vi "Pulse_Sequence_Global.vi"() -> ()   [LabVIEW 2021]
uses:
  Drivers/Arduino_Pulse_Generator/Configurate/Channel_Pulse_Stream.ctl
panel:
  out "Init outp register 2 (8-13)":bool[](array[boolean])
  out "Init outp register 1 (2-7)":bool[](array[boolean])
  out "Pulse sequence":T1[](array[typedef]) {"channel" min=2 max=13 step=1}
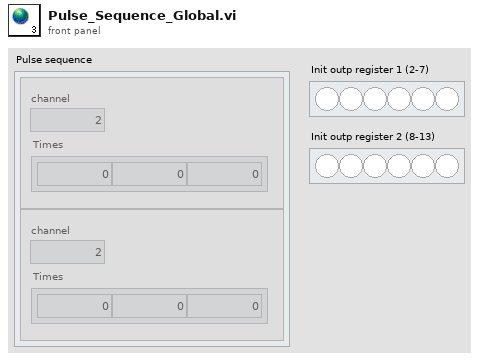
[diagram p1: front panel]
types:
  T1 = typedef "Channel_Pulse_Stream.ctl" = cluster{"Times":dbl[], "channel":u8}
diagram:
